vi "DataTree_LS1_back.vi"(0 "Arbre":refnum<vi>, 1 "Data Folder Path":path, 2 "ScanParamsIn":T1[](array[typedef]), 3 "VarParam":string, 5 "Date String":string="All" caption="Date String (yymmdd)", 9 "Session":i32=-1, 11 "error in (no error)":errorcluster, 12 "IncludeSubF":bool, 13 "Recheck Files":bool, 14 "KeyWord":string) -> (4 "Arbre Out":refnum<vi>, 6 "Headers Out":T1[](array[typedef]), 8 "FilesPath":path[](array[path]), 10 "Tous les tags":string[](array[string]), 15 "error out":errorcluster)   [LabVIEW 2019]
uses:
  Interface Class/ScanParams.ctl
  Interface Class/Interface.lvclass
panel:
  out "Tag Courbes":string[](array[string])
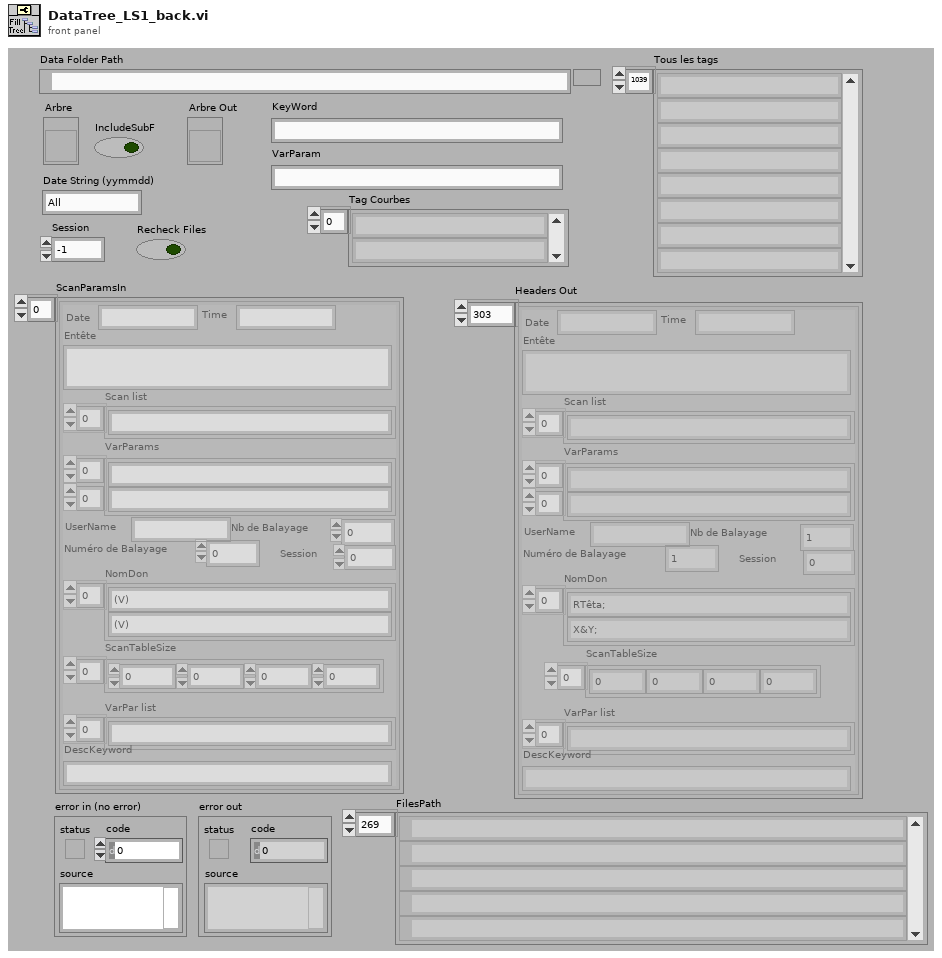
[diagram p1: front panel]
types:
  T1 = typedef "Interface.lvclass/ScanParams.ctl" = cluster{"Entête":string, "Scan list":string[], "NbCourbe":i32, "IndCourbe":i64, "NomDon":string[], "Session ":i32, "Date":string, "Time":string, "VarParams":string[][], "UserName":string, "ScanTableSize":i32[], "VarPar list":string[], "DescKeyword":string}
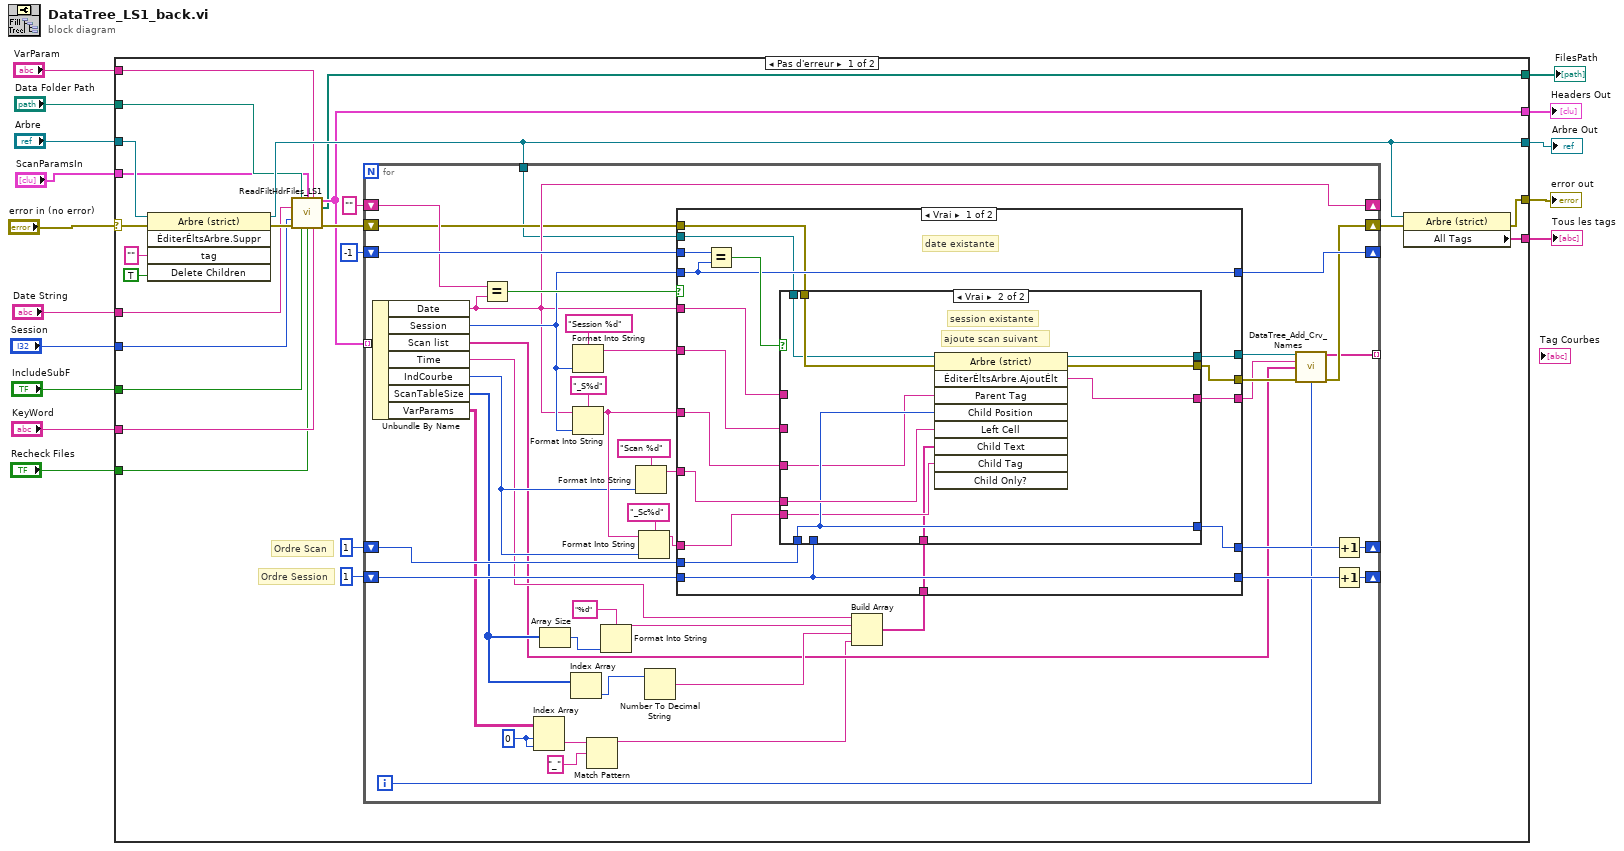
[diagram p0: block diagram]
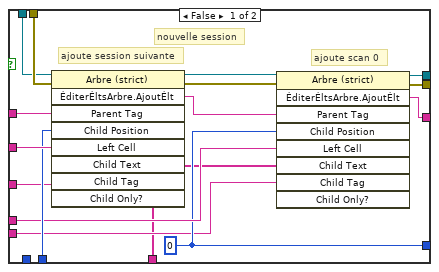
[diagram p2: hidden frame]
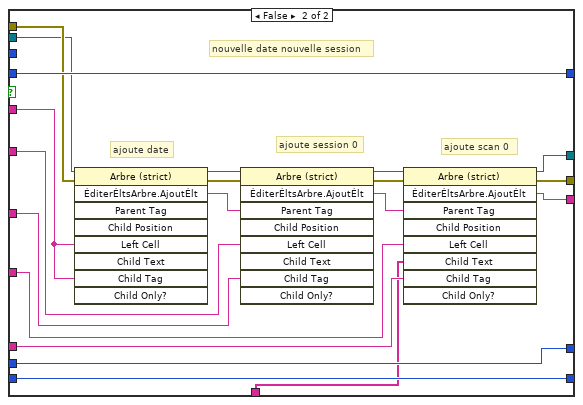
[diagram p3: hidden frame]
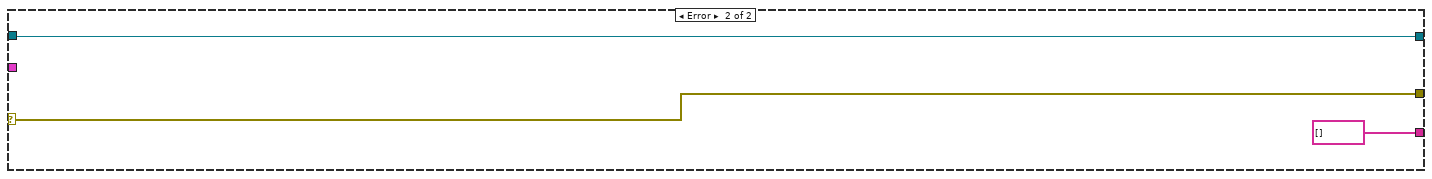
[diagram p4: hidden frame]
diagram:
  n1 = case shown="Pas d'erreur" "error in (no error)" {
    selector: "error in (no error)" -> [w30 w149]
    tunnel: [w39 string[] [] ("All Tags")] -> w15
    tunnel: [w32 w149] -> w13
    tunnel: [w22 _] -> w12
    tunnel: "Arbre" -> [w27 w147]
    tunnel: [w26 w147] -> w10
    tunnel: "Date String" -> [w25 _]
    tunnel: "Session" -> [w24 _]
    tunnel: "Data Folder Path" -> [w23 _]
    tunnel: "IncludeSubF" -> [w21 _]
    tunnel: "KeyWord" -> [w20 _]
    tunnel: "VarParam" -> [w19 _]
    tunnel: "ScanParamsIn" -> [w18 _]
    tunnel: "Recheck Files" -> [w17 _]
    tunnel: [w16 _] -> w1
    frame No Error {
      # "Ordre Scan"
      # "Ordre Session"
      n2 = invoke on="Nœud de méthode" class="Arbre (strict)" method="ÉditerÉltsArbre.Suppr"(reference=w27, error in=w30, "tag"="" ("Tag"), "Delete Children"=TRUE ("Supprimer les enfants ?")) -> (reference out=w26:refnum<vi>, error out=w29:errorcluster)  [unwired: 1 in, 3 out]
      n3 = call "ReadFiltHdrFiles_LS1.vi"("Data Folder Path"=w23, "ScanParamsIn"=w18, "VarParam"=w19, "Date String"=w25, "Session"=w24, "error in (no error)"=w29, "IncludeSubF"=w21, "Recheck Files"=w17, "KeyWord"=w20) -> ("ScanParamsOut"=w22:T1[], "FilesPath"=w16:path[], "error out"=w33:errorcluster)  [unwired: 4 in]
      n4 = for {
        tunnel: w22 -> [w83] mode=indexing
        shift-right: [w66] -> _
        shift-left: "" ("Date") -> [w74]
        shift-right: [w81] -> _
        shift-left: -1 ("Session") -> [w80]
        shift-right: [w79] -> _
        shift-left: 1 ("Session") -> [w75]
        shift-right: [w76] -> _
        shift-left: 1 ("Position de l'enfant") -> [w78]
        shift-right: [w61] -> w34
        shift-left: w33 -> [w63]
        tunnel: w26 -> [w57]
        tunnel: [w56] -> _ mode=indexing
        i -> [w46]
        w42 = 0 ("indice (ligne)")
        n5 = Unbundle By Name(w83) -> ("Date"=w66:string, "Session"=w67:i32, "Scan list"=w45:string[], "Time"=w50:string, "IndCourbe"=w54:i64, "ScanTableSize"=w53:i32[], "VarParams"=w41:string[][])
        n6 = Equal?(x=w74, y=w66) -> (x = y?=w82:bool)
        n7 = Index Array(array=w41, index (row)=w42, index (col)=w42) -> (element=w44:string)
        n8 = Array Size(array=w53) -> (size(s)=w52:i32)
        n9 = Index Array(array=w53) -> (element=w55:i32)  [unwired: 1 in]
        n10 = Format Into String(format string="Session %d" ("chaîne de format"), w67) -> (resulting string=w64:string)  [unwired: 2 in, 1 out]
        n11 = Format Into String(format string="_S%d" ("chaîne de format"), initial string=w66, w67) -> (resulting string=w65:string)  [unwired: 1 in, 1 out]
        n12 = Match Pattern(string=w44, regular expression="_" ("expression régulière")) -> (before substring=w40:string)  [unwired: 1 in, 3 out]
        n13 = Format Into String(format string="%d" ("chaîne de format"), w52) -> (resulting string=w49:string)  [unwired: 2 in, 1 out]
        n14 = Format Into String(format string="Scan %d" ("chaîne de format"), w54) -> (resulting string=w71:string)  [unwired: 2 in, 1 out]
        n15 = Format Into String(format string="_Sc%d" ("chaîne de format"), initial string=w65, w54) -> (resulting string=w70:string)  [unwired: 1 in, 1 out]
        n16 = Number To Decimal String(number=w55) -> (decimal integer string=w48:string)  [unwired: 1 in]
        n17 = Build Array(w50, w49, w48, w40) -> (w47:string[])
        n18 = case shown="Vrai" w82 {
          tunnel: w66 -> [w97 w144]
          tunnel: w67 -> [w90 w145]
          tunnel: [w90 w145] -> w81
          tunnel: w80 -> [w91 _]
          tunnel: w75 -> [w99 w133]
          tunnel: [w98 w133] -> w62
          tunnel: w78 -> [w96 w143]
          tunnel: [w96 w143] -> w77
          tunnel: w71 -> [w95 w139]
          tunnel: w70 -> [w94 w132]
          tunnel: w65 -> [w93 w137]
          tunnel: w64 -> [w92 w138]
          tunnel: w63 -> [w88 w136]
          tunnel: [w89 w135] -> w59
          tunnel: [w87 w134] -> w60
          tunnel: w57 -> [w86 w131]
          tunnel: [w85 w128] -> w58
          tunnel: w47 -> [w84 w127]
          frame True {
            # "date existante"
            n19 = Equal?(x=w91, y=w90) -> (x = y?=w100:bool)
            n20 = case shown="Vrai" w100 {
              tunnel: w92 -> [w115 _]
              tunnel: w97 -> [w116 _]
              tunnel: w99 -> [_ w125]
              tunnel: [w110 w125] -> w98
              tunnel: w96 -> [w114 _]
              tunnel: [w108 w121] -> w87
              tunnel: w93 -> [w109 w124]
              tunnel: w95 -> [w111 w126]
              tunnel: w94 -> [w105 w123]
              tunnel: [w107 w122] -> w89
              tunnel: w88 -> [w106 w120]
              tunnel: w86 -> [w104 w119]
              tunnel: [w102 w118] -> w85
              tunnel: w84 -> [w101 w117]
              frame False {
                w110 = 0 ("Session")
                # "ajoute scan 0"
                # "ajoute session suivante"
                # "nouvelle session"
                n21 = invoke on="Nœud de méthode" class="Arbre (strict)" method="ÉditerÉltsArbre.AjoutÉlt"(reference=w104, error in=w106, "Parent Tag"=w116, "Child Position"=w114, "Left Cell"=w115, "Child Tag"=w109) -> (reference out=w103:refnum<vi>, error out=w113:errorcluster, "Edit Tree Items:Add Item"=w112:string)  [unwired: 3 in, 6 out]
                n22 = invoke on="Nœud de méthode" class="Arbre (strict)" method="ÉditerÉltsArbre.AjoutÉlt"(reference=w103, error in=w113, "Parent Tag"=w112, "Child Position"=w110, "Left Cell"=w111, "Child Text"=w101, "Child Tag"=w105) -> (reference out=w102:refnum<vi>, error out=w108:errorcluster, "Edit Tree Items:Add Item"=w107:string)  [unwired: 2 in, 6 out]
              }
              frame True {
                # "ajoute scan suivant"
                # "session existante"
                n23 = invoke on="Nœud de méthode" class="Arbre (strict)" method="ÉditerÉltsArbre.AjoutÉlt"(reference=w119, error in=w120, "Parent Tag"=w124, "Child Position"=w125, "Left Cell"=w126, "Child Text"=w117, "Child Tag"=w123) -> (reference out=w118:refnum<vi>, error out=w121:errorcluster, "Edit Tree Items:Add Item"=w122:string)  [unwired: 2 in, 6 out]
              }
            }
          }
          frame False {
            # "ajoute date"
            # "ajoute scan 0"
            # "ajoute session 0"
            # "nouvelle date nouvelle session"
            n24 = invoke on="Nœud de méthode" class="Arbre (strict)" method="ÉditerÉltsArbre.AjoutÉlt"(reference=w131, error in=w136, "Left Cell"=w144, "Child Tag"=w144) -> (reference out=w130:refnum<vi>, error out=w146:errorcluster, "Edit Tree Items:Add Item"=w140:string)  [unwired: 5 in, 6 out]
            n25 = invoke on="Nœud de méthode" class="Arbre (strict)" method="ÉditerÉltsArbre.AjoutÉlt"(reference=w130, error in=w146, "Parent Tag"=w140, "Left Cell"=w138, "Child Tag"=w137) -> (reference out=w129:refnum<vi>, error out=w142:errorcluster, "Edit Tree Items:Add Item"=w141:string)  [unwired: 4 in, 6 out]
            n26 = invoke on="Nœud de méthode" class="Arbre (strict)" method="ÉditerÉltsArbre.AjoutÉlt"(reference=w129, error in=w142, "Parent Tag"=w141, "Left Cell"=w139, "Child Text"=w127, "Child Tag"=w132) -> (reference out=w128:refnum<vi>, error out=w134:errorcluster, "Edit Tree Items:Add Item"=w135:string)  [unwired: 3 in, 6 out]
          }
        }
        n27 = call "DataTree_Add_Crv_Names.vi"("référence"=w58, "Parent Name"=w59, "Scan list"=w45, "Entrée d'erreur"=w60, "FileIndex"=w46) -> ("Tag Courbes"=w56:string[], "Sortie d'erreur"=w61:errorcluster)  [unwired: 9 in]
        n28 = Increment(x=w62) -> (x+1=w79:i32)
        n29 = Increment(x=w77) -> (x+1=w76:i32)
      }
      n30 = property on="Nœud de propriété" class="Arbre (strict)"(reference=w26, error in=w34) -> (error out=w32:errorcluster, "All Tags"=w39:string[])  [unwired: 1 out]
    }
    frame Error {
    }
  }
  "Tous les tags" <- w15
  "error out" <- w13
  "Headers Out" <- w12
  "Arbre Out" <- w10
  "FilesPath" <- w1
